vi "DAQ Done.vi"(0 "Module Name":string, 1 "Event Number":i32) -> ()   [LabVIEW 2009]
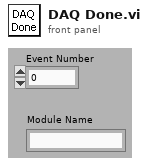
[diagram p1: front panel]
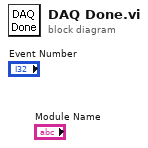
[diagram p0: block diagram]
diagram:
